vi "Decode Single Tag.vi"(8 "Error In":errorcluster, 11 "PicoQuant Tag":T1 {"TagType" format="%.0x"}) -> (0 "Error Out":errorcluster, 3 "Variant":variant)   [LabVIEW 2021, in "PTU Files.lvlib"]
uses:
  PTU Files.lvlib
  PicoQuant Header Tag.ctl
  PicoQuant Tag Type.ctl
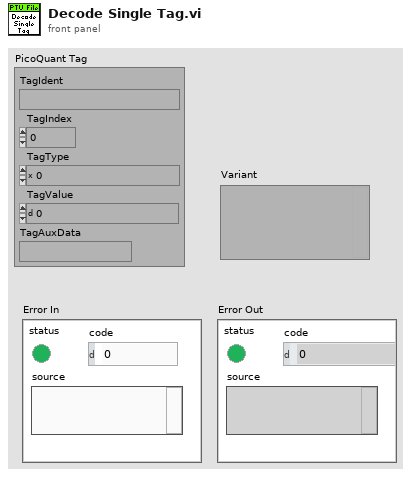
[diagram p1: front panel]
types:
  T1 = typedef "PTU Files.lvlib/PicoQuant Header Tag.ctl" = cluster{"TagIdent":string, "TagIndex":i32, "TagType":i32, "TagValue":i64, "TagAuxData":string}
  T2 = typedef "PTU Files.lvlib/PicoQuant Tag Type.ctl" = i32
  T3 = enum16{"big-endian, network order", "native, host order", "little-endian"}
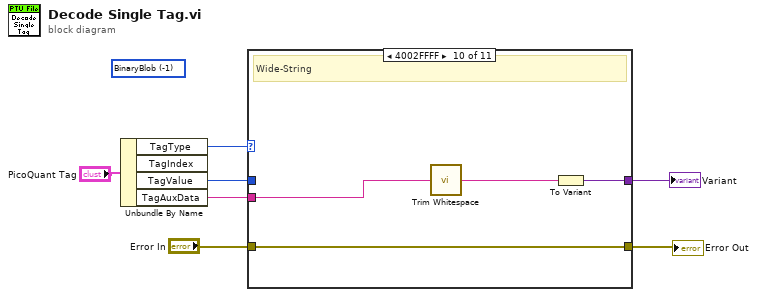
[diagram p0: block diagram]
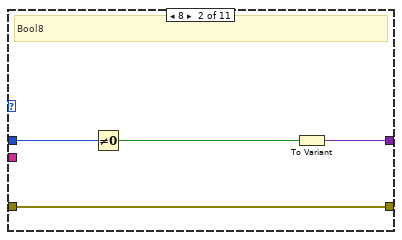
[diagram p3: hidden frame]
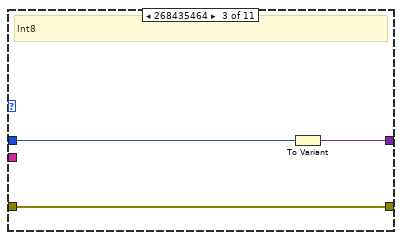
[diagram p4: hidden frame]
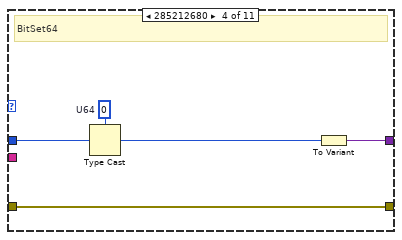
[diagram p5: hidden frame]
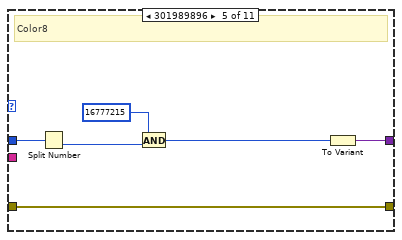
[diagram p6: hidden frame]
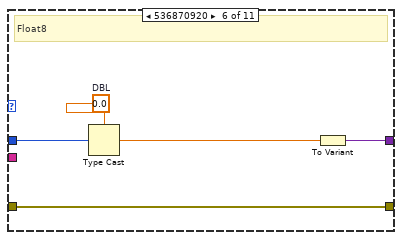
[diagram p7: hidden frame]
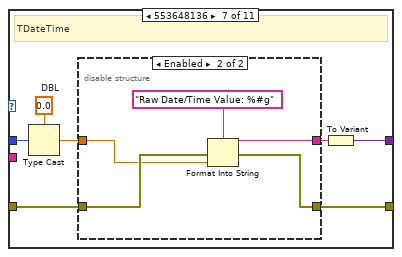
[diagram p8: hidden frame]
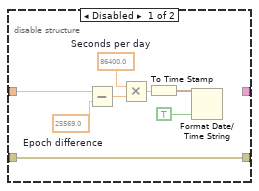
[diagram p9: hidden frame]
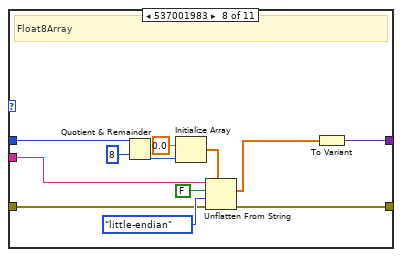
[diagram p10: hidden frame]
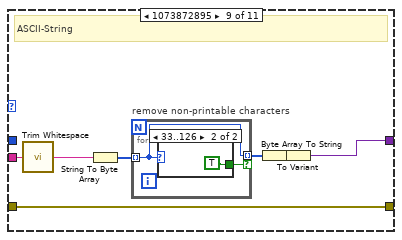
[diagram p11: hidden frame]
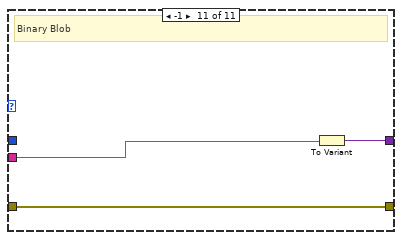
[diagram p13: hidden frame]
diagram:
  (unwired) T2 -1 items=["Empty8"=-65528, "Bool8"=8, "Int8"=268435464, "BitSet64"=285212680, "Color8"=301989896, "Float8"=536870920, "TDateTime"=553648136, "Float8Array"=537001983, "ASCII-String"=1073872895, "Wide-String"=1073938431, "BinaryBlob"=-1] ("Tag Type")
  n1 = Unbundle By Name("PicoQuant Tag") -> ("TagType"=w5:i32, "TagValue"=w4:i64, "TagAuxData"=w3:string)  [unwired: 1 out]
  n2 = case shown="4002FFFF" w5 {
    tunnel: w4 -> [_ w12 w15 w20 w25 w31 w38 w62 _ _ _]
    tunnel: [_ w10 w14 w19 w26 w30 w37 w63 w70 w77 w80] -> w7
    tunnel: w3 -> [_ _ _ _ _ _ _ w56 w68 w75 w78]
    tunnel: "Error In" -> [w8 w9 w13 w16 w21 w27 w33 w54 w69 w76 w79]
    tunnel: [w8 w9 w13 w16 w21 w27 w32 w52 w69 w76 w79] -> w1
    frame -65528, Default {
      # "Empty8"
    }
    frame 8 {
      # "Bool8"
      n3 = Not Equal To 0?(x=w12) -> (x != 0?=w11:bool)
      n4 = To Variant(anything=w11) -> (Variant=w10:variant)
    }
    frame 268435464 {
      # "Int8"
      n5 = To Variant(anything=w15) -> (Variant=w14:variant)
    }
    frame 285212680 {
      w17 = u64 0  # U64
      # "BitSet64"
      n6 = Type Cast(type=w17, x=w20) -> (*(type *) &x=w18:u64)
      n7 = To Variant(anything=w18) -> (Variant=w19:variant)
    }
    frame 301989896 {
      # "Color8"
      n8 = Split Number(x=w25) -> (lo(x)=w23:u32)  [unwired: 1 out]
      n9 = And(x=u32 16777215 ("y"), y=w23) -> (x .and. y?=w24:u32)
      n10 = To Variant(anything=w24) -> (Variant=w26:variant)
    }
    frame 536870920 {
      w28 = 0.0  # DBL
      # "Float8"
      n11 = Type Cast(type=w28, x=w31) -> (*(type *) &x=w29:dbl)
      n12 = To Variant(anything=w29) -> (Variant=w30:variant)
    }
    frame 553648136 {
      w36 = 0.0  # DBL
      # "TDateTime"
      n13 = Type Cast(type=w36, x=w38) -> (*(type *) &x=w35:dbl)
      n14 = disable-structure shown="Enabled" {
        disable-tunnel: w35 -> [w40 w47]
        disable-tunnel: [_ w50] -> w34
        disable-tunnel: w33 -> [w39 w49]
        disable-tunnel: [w39 w48] -> w32
        frame Disabled {
          w44 = 86400.0  # Seconds per day
          w46 = 25569.0  # Epoch difference
          n15 = Subtract(x=w40, y=w46) -> (x-y=w45:dbl)
          n16 = Multiply(x=w44, y=w45) -> (x*y=w43:dbl)
          n17 = To Time Stamp(1:w43) -> (0:w42:timestamp)
          n18 = Format Date/Time String(seconds (now)=w42, UTC format=TRUE) -> ()  [unwired: 1 in, 1 out]
        }
        frame Enabled {
          n19 = Format Into String(format string="Raw Date/Time Value: %#g" ("date/time string"), error in=w49, w47) -> (resulting string=w50:string, error out=w48:errorcluster)  [unwired: 1 in]
        }
      }
      n20 = To Variant(anything=w34) -> (Variant=w37:variant)
    }
    frame 537001983 {
      # "Float8Array"
      n21 = Quotient & Remainder(x=w62, y=i64 8) -> (floor(x/y)=w57:i64)  [unwired: 1 out]
      n22 = Initialize Array(0.0, w57) -> (w59:dbl[])
      n23 = Unflatten From String(type=w59, binary string=w56, data includes array or string size? (T)=FALSE, byte order (0:big-endian, network order)=T3."little-endian", error in (no error)=w54) -> (value=w53:dbl[], error out=w52:errorcluster)  [unwired: 1 out]
      n24 = To Variant(anything=w53) -> (Variant=w63:variant)
    }
    frame 1073872895 {
      # "ASCII-String"
      n25 = call <vilib>:"Trim Whitespace.vi"("string"=w68) -> ("trimmed string"=w67:string)  [unwired: 1 in]
      n26 = String To Byte Array(string=w67) -> (unsigned byte array=w66:u8[])
      n27 = for "remove non-printable characters" {
        tunnel: w66 -> [w72] mode=indexing
        tunnel: [w72] -> w65 mode=indexing if=w71
        n28 = case shown="33..126" w72 {
          tunnel: [_ TRUE] -> w71
          frame 0, Default {
          }
          frame 33..126 {
          }
        }
      }
      n29 = Byte Array To String(unsigned byte array=w65) -> (string=w64:string)
      n30 = To Variant(anything=w64) -> (Variant=w70:variant)
    }
    frame 1073938431 {
      # "Wide-String"
      n31 = call <vilib>:"Trim Whitespace.vi"("string"=w75) -> ("trimmed string"=w74:string)  [unwired: 1 in]
      n32 = To Variant(anything=w74) -> (Variant=w77:variant)
    }
    frame -1 {
      # "Binary Blob"
      n33 = To Variant(anything=w78) -> (Variant=w80:variant)
    }
  }
  "Variant" <- w7
  "Error Out" <- w1
